vi "Fill.vi"(8 "error in (no error)":errorcluster, 10 "Color":refnum<class "Color.lvclass">, 11 "senseHatDisplay in":refnum<class "RPI.SenseHat.Display.lvclass">) -> (0 "error out":errorcluster, 3 "senseHatDisplay out":refnum<class "RPI.SenseHat.Display.lvclass">)   [LabVIEW 2020, in "RPI.SenseHat.Display.lvlib" / "RPI.SenseHat.Display.lvclass"]
doc: "Fills the screen of the given color.\n\nNote: Requires a call to Update to affect the physical screen."
uses:
  RPI.SenseHat.Display.lvclass
  Color/Color.lvclass
  RPI.SenseHat.Display.lvclass/RPI.SenseHat.Display.ctl
  Image/Image.lvclass
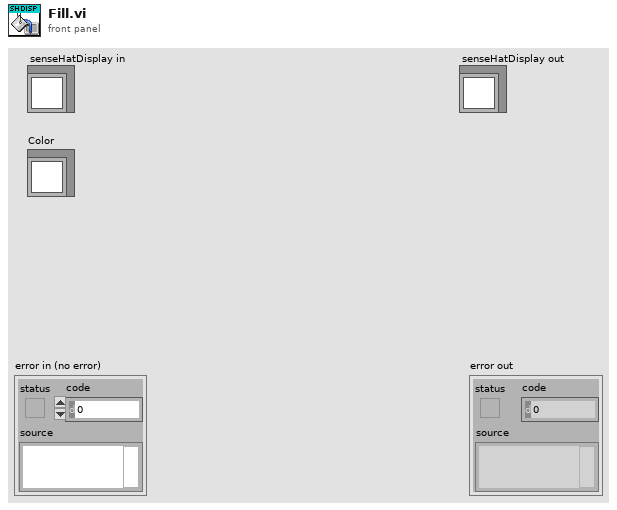
[diagram p1: front panel]
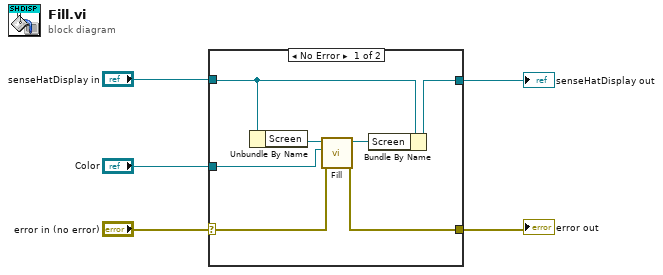
[diagram p0: block diagram]
diagram:
  n1 = case shown="No Error" "error in (no error)" {
    selector: "error in (no error)" -> [w8 w14]
    tunnel: [w7 w14] -> w4
    tunnel: [w10 w13] -> w2
    tunnel: "senseHatDisplay in" -> [w11 w13]
    tunnel: "Color" -> [w6 _]
    frame No Error {
      n2 = Unbundle By Name(w11) -> ("Screen"=w12:refnum<class "Image.lvclass">)
      n3 = call "Fill.vi"("error in (no error)"=w8, "Color"=w6, "Image in"=w12) -> ("error out"=w7:errorcluster, "Image out"=w9:refnum<class "Image.lvclass">)  [unwired: 7 in]
      n4 = Bundle By Name(cluster=w11, "Screen"=w9) -> (w10:refnum<class "RPI.SenseHat.Display.lvclass">)
    }
    frame Error {
    }
  }
  "error out" <- w4
  "senseHatDisplay out" <- w2
